vi "Load Project From File.vi"(8 "error in":errorcluster, 11 "Project Path":path) -> (0 "error out":errorcluster, 1 "Continue?":bool, 3 "Project out":refnum<class "Project.lvclass">)   [LabVIEW 2020, in "Panther Dashboard.lvlib" / "Project.lvclass"]
uses:
  Project.lvclass
  C:/GitClones/PantherDashboard/src/LabVIEW/Panther Dashboard/Class/LabVIEWItem/LabVIEWItem.lvclass
  LabVIEWItem/LabVIEWItem.lvclass/LabVIEWItem.ctl
  Project.lvclass/Project.ctl
  Library/Library.lvclass/Library.ctl
  LabVIEWItem/Read Item Path.vi
  Library/Write Library Ref.vi
  Read Target Name.vi
  Read Libraries.vi
  Read Target App Ins Ref.vi
  Write Libraries.vi
  LabVIEWItem/Write Item Path.vi
  Library/Library.lvclass
  Panther Dashboard/Panther Dashboard.lvlib
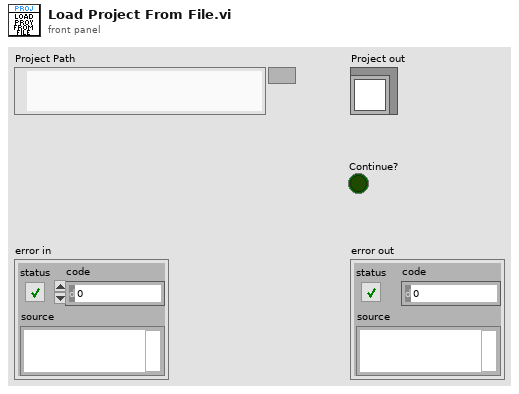
[diagram p1: front panel]
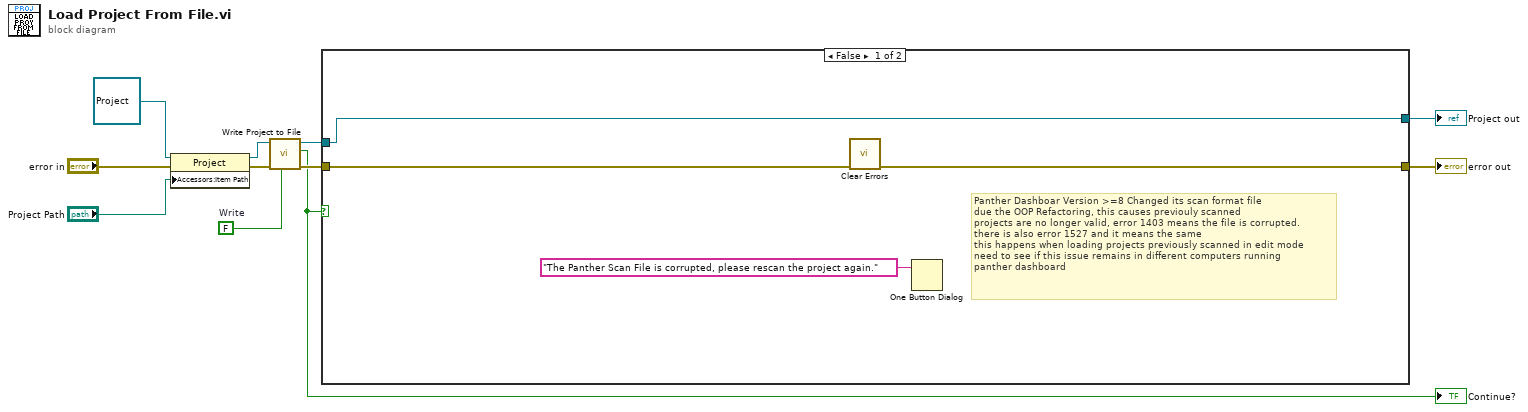
[diagram p0: block diagram]
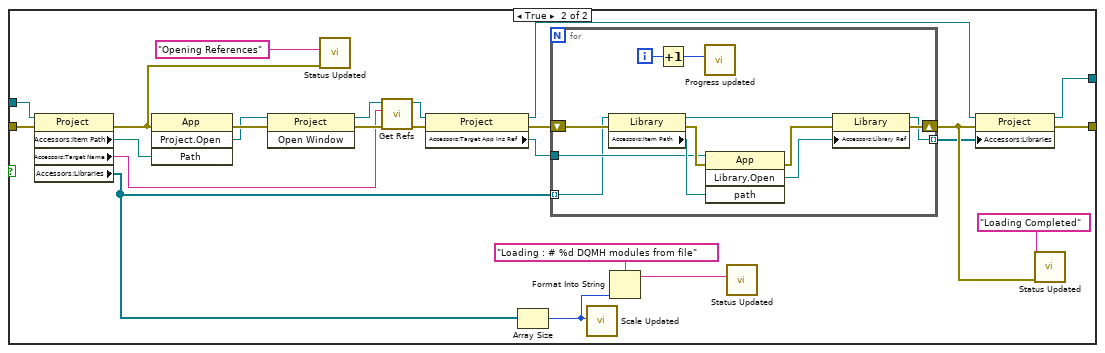
[diagram p2: hidden frame]
diagram:
  w6 = FALSE  # Write
  n1 = property class="Project"(reference=refnum<class "Project.lvclass"> refnum ("Project In"), error in="error in", "Accessors:Item Path"="Project Path") -> (reference out=w3:refnum<class "Project.lvclass">, error out=w8:errorcluster)
  n2 = call "Write Project to File.vi"("Write"=w6, "error in"=w8, "Project In"=w3) -> ("error out"=w9:errorcluster, "Continue?"=w1:bool, "Project Out"=w4:refnum<class "Project.lvclass">)  [unwired: 6 in]
  "Continue?" <- w1
  n3 = case shown="False" w1 {
    tunnel: [w13 w36] -> w11
    tunnel: w9 -> [w14 w35]
    tunnel: [w15 w19] -> w7
    tunnel: w4 -> [w15 w18]
    frame False {
      # "Panther Dashboar Version >=8 Changed its scan format file\ndue the OOP Refactoring, this causes previouly scanned \nprojects are no longer valid, error 1403 means the file is corrupted.\nthere is also error 1527 and it means the same\nthis happens when loading projects previously scanned in edit mode\nneed to see if this issue remains in different computers running\npanther dashboard"
      n4 = call <vilib>:"Clear Errors.vi"("error in (no error)"=w14) -> ("error out"=w13:errorcluster)  [unwired: 5 in, 1 out]
      n5 = One Button Dialog(message="The Panther Scan File is corrupted, please rescan the project again." ("Status")) -> ()  [unwired: 1 in, 1 out]
    }
    frame True {
      n6 = property class="Project"(reference=w18, error in=w35) -> (error out=w32:errorcluster, "Accessors:Item Path"=w21:path, "Accessors:Target Name"=w22:string, "Accessors:Libraries"=w17:refnum<class "Library.lvclass">[])  [unwired: 1 out]
      n7 = invoke class="App" method="Project.Open"(error in=w32, "Path"=w21) -> (error out=w39:errorcluster, "Project:Open"=w30:refnum<vi>)  [unwired: 2 in, 2 out]
      n8 = invoke class="Project" method="Open Window"(reference=w30, error in=w39) -> (reference out=w31:refnum<vi>, error out=w34:errorcluster)  [unwired: 1 in, 1 out]
      n9 = call "Status Updated.vi"("error in (no error)"=w32, "Status"="Opening References") -> ()  [unwired: 9 in, 1 out]
      n10 = call "Get Refs.vi"("error in"=w34, "Target Selection"=w22, "Project in"=w31) -> ("error out"=w38:errorcluster, "Project"=w24:refnum<class "Project.lvclass">)  [unwired: 7 in]
      n11 = property class="Project"(reference=w24, error in=w38) -> (reference out=w16:refnum<class "Project.lvclass">, error out=w37:errorcluster, "Accessors:Target App Ins Ref"=w23:refnum<vi>)
      n12 = Array Size(array=w17) -> (size(s)=w26:i32)
      n13 = for {
        shift-right: [w48] -> w33
        shift-left: w37 -> [w51]
        tunnel: w23 -> [w44]
        tunnel: [w42] -> w20 mode=indexing
        tunnel: w17 -> [w40] mode=indexing
        i -> [w47]
        n14 = property class="Library"(reference=w40, error in=w51) -> (reference out=w43:refnum<class "Library.lvclass">, error out=w50:errorcluster, "Accessors:Item Path"=w45:path)
        n15 = Increment(x=w47) -> (x+1=w46:i32)
        n16 = call "Progress updated.vi"("Progress"=w46) -> ()  [unwired: 10 in, 1 out]
        n17 = invoke class="App" method="Library.Open"(reference=w44, error in=w50, "path"=w45) -> (error out=w49:errorcluster, "Open Library"=w41:refnum<vi>)  [unwired: 1 in, 2 out]
        n18 = property class="Library"(reference=w43, error in=w49, "Accessors:Library Ref"=w41) -> (reference out=w42:refnum<class "Library.lvclass">, error out=w48:errorcluster)
      }
      n19 = call "Scale Updated.vi"("Scale Max"=w26) -> ()  [unwired: 10 in, 1 out]
      n20 = Format Into String(format string="Loading : # %d DQMH modules from file", w26) -> (resulting string=w28:string)  [unwired: 2 in, 1 out]
      n21 = call "Status Updated.vi"("Status"=w28) -> ()  [unwired: 10 in, 1 out]
      n22 = property class="Project"(reference=w16, error in=w33, "Accessors:Libraries"=w20) -> (reference out=w19:refnum<class "Project.lvclass">, error out=w36:errorcluster)
      n23 = call "Status Updated.vi"("error in (no error)"=w33, "Status"="Loading Completed") -> ()  [unwired: 9 in, 1 out]
    }
  }
  "error out" <- w11
  "Project out" <- w7
